vi "FOUR_U8_TO_FLOAT.vi"(1 "接收数据4*U8":u8[](array[numeric])) -> (0 "浮点结果":dbl)   [LabVIEW 2014]
panel:
  # "四个字节高八位为整数位 低八位为小数位 经过转化为浮点数"
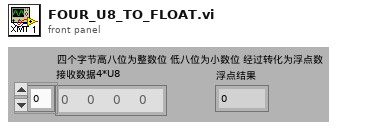
[diagram p1: front panel]
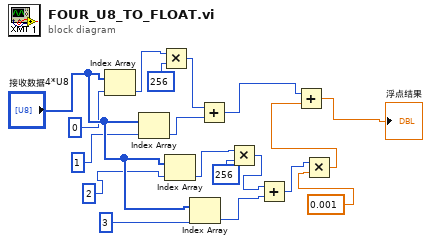
[diagram p0: block diagram]
diagram:
  n1 = Index Array(array="接收数据4*U8", index=0) -> (element=w13:u8)
  n2 = Index Array(array="接收数据4*U8", index=1) -> (element=w12:u8)
  n3 = Multiply(x=w13, y=256) -> (x*y=w8:i32)
  n4 = Index Array(array="接收数据4*U8", index=2) -> (element=w11:u8)
  n5 = Index Array(array="接收数据4*U8", index=3) -> (element=w10:u8)
  n6 = Add(x=w8, y=w12) -> (x+y=w3:i32)
  n7 = Multiply(x=w11, y=256) -> (x*y=w6:i32)
  n8 = Add(x=w6, y=w10) -> (x+y=w5:i32)
  n9 = Multiply(x=w5, y=0.001) -> (x*y=w2:dbl)
  n10 = Add(x=w3, y=w2) -> (x+y=→"浮点结果":dbl)
